vi "Get VF Setpoints.vi"(10 "Per-Unitized VF Voltage Setpoint":dbl, 11 "Resynchronization in":refnum<class "Resynchronization.lvclass">) -> (1 "VF Frequency Setpoint":dbl, 2 "VF Voltage Setpoint":dbl, 3 "Resynchronization out":refnum<class "Resynchronization.lvclass">)   [LabVIEW 2018, in "Resynchronization Actor.lvlib" / "Resynchronization.lvclass"]
uses:
  Resynchronization.lvclass
  C:/Users/Administrator/Desktop/LabVIEW EMS/EMS Generic Actor/EMS Generic/EMS Generic.lvclass
  EMS Generic Actor/EMS Generic/EMS Generic.lvclass/EMS Generic.ctl
  EMS Generic Actor/EMS Generic/EMS Generic.lvclass
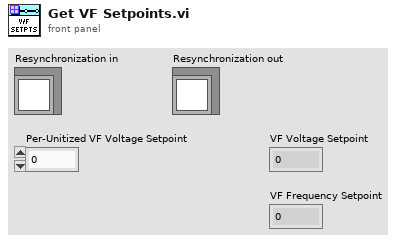
[diagram p1: front panel]
types:
  T1 = typedef "EMS Generic Actor.lvlib/EMS Generic.lvclass/Global Configuration.ctl" = cluster{"Microgrid ID":u8, "VF Device ID":T2, "Ongrid VF Priority":T2[], "Offgrid VF Priority":T2[], "AutoSwap Offgrid VF":u32, "AutoSwap Offgrid VF Delay (sec)":dbl, "AutoSwap Resynch VF":u32, "PCC Device ID":T2, "Device ID Array":T2[], "Nominal Voltage":dbl, "Nominal Frequency":dbl, "Resynch Timeout (sec)":dbl, "Island VF Activate Timeout (sec)":dbl, "Island PCC Target Power (kW)":dbl, "Island PCC Target Power Timeout (sec)":dbl, "Island Grid Settle Time (sec)":dbl, "Island PCC Failure Timeout (sec)":dbl, "Activation Devices Present Timeout (sec)":dbl, "Activation Devices Activated Timeout (sec)":dbl, "Blackstart VF GenMode Wait (sec)":dbl, "Blackstart VF DERCtrl Wait (sec)":dbl, "Blackstart Success Wait (sec)":dbl, "OnGrid Optimization Delay (sec)":dbl, "OffGrid Optimization Delay (sec)":dbl, "Resynch Frequency (Hz)":dbl, "Optimization Path":string}
  T2 = typedef "CSEISMIC DDS.lvlib/CSEISMIC DDS.lvclass/DeviceID.ctl" = string
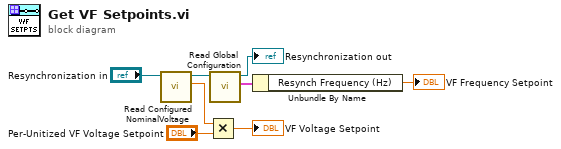
[diagram p0: block diagram]
diagram:
  n1 = call "Read Configured NominalVoltage.vi"("EMS Generic in"="Resynchronization in") -> ("NominalVoltage"=w7:dbl, "EMS Generic out"=w4:refnum<class "Resynchronization.lvclass">)  [unwired: 8 in, 1 out]
  n2 = Multiply(x=w7, y="Per-Unitized VF Voltage Setpoint") -> (x*y=→"VF Voltage Setpoint":dbl)
  n3 = call "Read Global Configuration.vi"("EMS Generic in"=w4) -> ("Global Configuration"=w2:T1, "dup EMS Generic out"=→"Resynchronization out":refnum<class "Resynchronization.lvclass">)  [unwired: 8 in, 1 out]
  n4 = Unbundle By Name(w2) -> ("Resynch Frequency (Hz)"=→"VF Frequency Setpoint":dbl)
